vi "Vision Research Phantom Series PhCon PhSetDllsOption.vi"(0 "optionSelector":T1 items=["DO_IGNORECAMERAS"=1], 5 "Error In (no error)":errorcluster) -> (14 "pVal [out]":i32, 19 "Error Out":errorcluster)   [LabVIEW 2013, in "VRI.lvlib"]
doc: "PhSetDllsOption\nHRESULT PhSetDllsOption(UINT optionSelector, PVOID pValue)\n\nParameters\noptionSelector [in]\n Value indicating the option to be set. \npValue [out]\n Buffer containing the value to be set. \n\nReturn Value\nThe function returns ERR_Ok in case of success or an error code, otherwise. To get extended error information call PhGetErrorMessage.\n\nRemarks\nSets various user options regarding Phantom dlls use. This function must be called before PhRegisterClientEx.\n\nRequired Header\nPhCon.h"
uses:
  VRI.lvlib
  _Type Defs/PhCon PhSetDllsOptions.ctl
  Phantom DLLs/PhCon.Dll
panel:
  # "For instructions on the use of this VI, press Ctrl+H to display the help window and move the mouse over the icon, controls, and indicators"
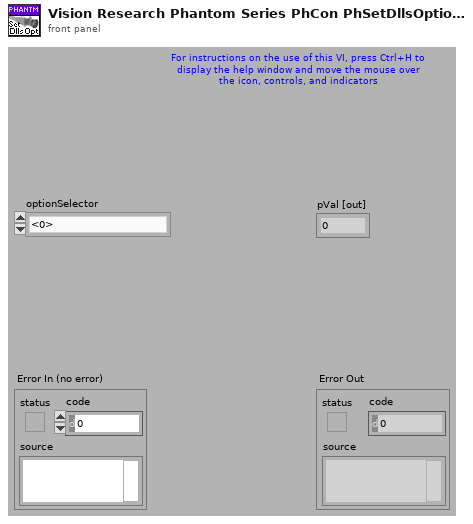
[diagram p1: front panel]
types:
  T1 = typedef "VRI.lvlib/PhCon PhSetDllsOptions.ctl" = u16
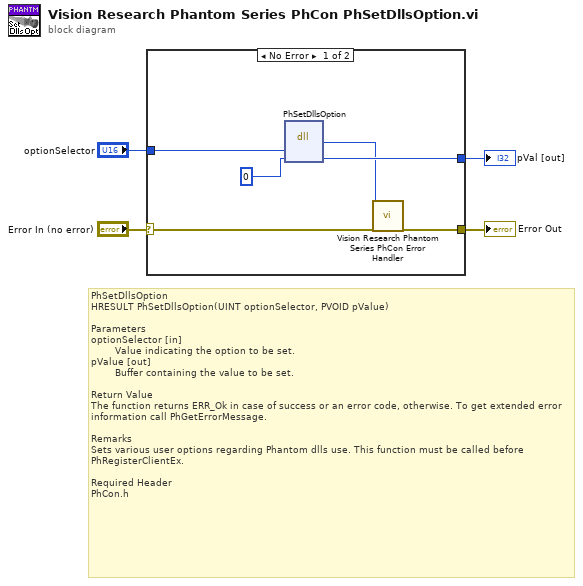
[diagram p0: block diagram]
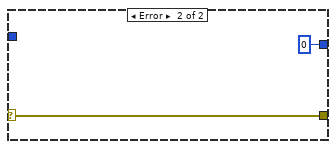
[diagram p2: hidden frame]
diagram:
  # "PhSetDllsOption\nHRESULT PhSetDllsOption(UINT optionSelector, PVOID pValue)\n\nParameters\noptionSelector [in]\n\t       Value indicating the option to be set. \npValue [out]\n        Buffer containing the value to be set. \n\nReturn Value\nThe function returns ERR_Ok in case of success or an error code, otherwise. To get extended error information call PhGetErrorMessage.\n\nRemarks\nSets various user options regarding Phantom dlls use. This function must be called before PhRegisterClientEx.\n\nRequired Header\nPhCon.h"
  n1 = case shown="No Error" "Error In (no error)" {
    selector: "Error In (no error)" -> [w10 w12]
    tunnel: [w9 w12] -> w3
    tunnel: "optionSelector" -> [w8 _]
    tunnel: [w7 0 ("pVal")] -> w1
    frame No Error {
      n2 = dll-call lib="C:/Projects/SDK/64-bit/Vision Research Phantom Series Labview Driver/Phantom DLLs/PhCon.dll" fn="PhSetDllsOption"("optionSelector"=w8, "pVal"=0) -> ("HRESULT"=w6:i32, "pVal"=w7:i32)  [unwired: 3 in, 3 out]
      n3 = call "Vision Research Phantom Series PhCon Error Handler.vi"("ErrNo"=w6, "Error In (no error)"=w10) -> ("Error Out"=w9:errorcluster)  [unwired: 17 out]
    }
    frame Error {
    }
  }
  "Error Out" <- w3
  "pVal [out]" <- w1
